vi "_Create Base Folder.vi"(8 "Error In":errorcluster, 11 "Root Folder":path) -> (0 "Error Out":errorcluster, 3 "Base Folder":path)   [LabVIEW 2015, in "Logger.lvlib" / "File.lvlib"]
uses:
  File.lvlib
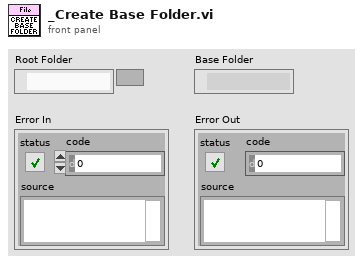
[diagram p1: front panel]
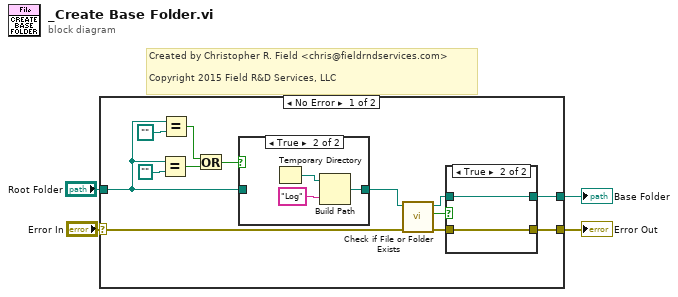
[diagram p0: block diagram]
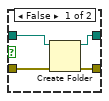
[diagram p2: hidden frame]
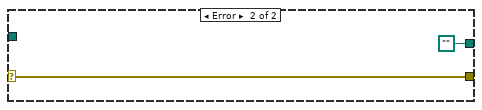
[diagram p4: hidden frame]
diagram:
  # "Created by Christopher R. Field <chris@fieldrndservices.com>\n\nCopyright 2015 Field R&D Services, LLC"
  n1 = case shown="No Error" "Error In" {
    selector: "Error In" -> [w10 w29]
    tunnel: "Root Folder" -> [w12 _]
    tunnel: [w6 path ""] -> w2
    tunnel: [w5 w29] -> w1
    frame No Error {
      n2 = Equal?(x=w12, y=path "") -> (x = y?=w14:bool)
      n3 = Equal?(x=w12, y=path "") -> (x = y?=w15:bool)
      n4 = Or(x=w15, y=w14) -> (x .or. y?=w13:bool)
      n5 = case shown="True" w13 {
        tunnel: [w24 w26] -> w11
        tunnel: w12 -> [w24 _]
        frame False {
        }
        frame True {
          n6 = Temporary Directory() -> (w25:path)
          n7 = Build Path(base path=w25, name or relative path="Log") -> (appended path=w26:path)
        }
      }
      n8 = call <vilib>:"Check if File or Folder Exists.vi"("error in (no error)"=w10, "path"=w11) -> ("error out"=w7:errorcluster, "file or folder exists?"=w9:bool, "dup path"=w8:path)  [unwired: 7 in]
      n9 = case shown="True" w9 {
        tunnel: w8 -> [w21 w23]
        tunnel: w7 -> [w20 w22]
        tunnel: [w19 w23] -> w6
        tunnel: [w18 w22] -> w5
        frame False {
          n10 = Create Folder(path (use dialog)=w21, error in=w20) -> (created path=w19:path, error out=w18:errorcluster)  [unwired: 1 in, 1 out]
        }
        frame True {
        }
      }
    }
    frame Error {
    }
  }
  "Base Folder" <- w2
  "Error Out" <- w1
